vi "Patrick-UTiLIA-RollingAverage.vi"(5 "Restart Avg":bool, 6 "Current Average":dbl=0.09818164425343229 format="%.5f", 7 "Rolling Avg Parameters":T1={"Rolling Avg mode"=enum."No Averaging", "# of averages"=10} {"# of averages" min=1}, 8 "Signal to Average":dbl[](array[numeric]) format="%.2f") -> (0 "averages completed":i16, 1 "Long-term Average":dbl=0.09818164425343229 format="%.5f", 2 "Chunk Fluctuations":dbl=0.00023658579987782333 format="%.3f", 3 "Chunk Average":dbl=0.09818164425343229 format="%.5f", 4 "averaging done":bool)   [LabVIEW 2013]
uses:
  <vilib>/Analysis/NI_AALBase.lvlib
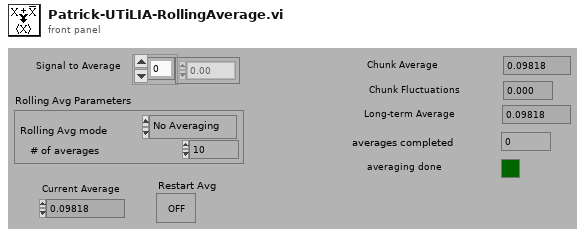
[diagram p1: front panel]
types:
  T1 = cluster{"Rolling Avg mode":enum16{"No Averaging", "Linear", "Exponential"}, "# of averages":u32}
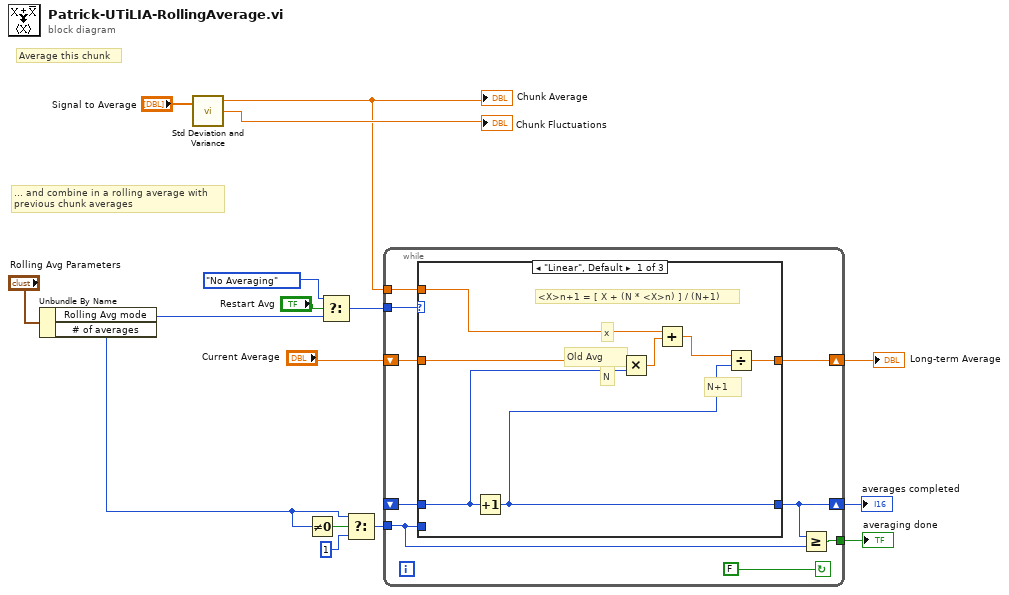
[diagram p0: block diagram]
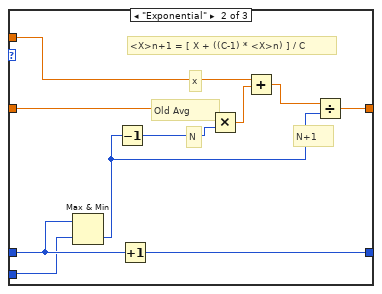
[diagram p2: hidden frame]
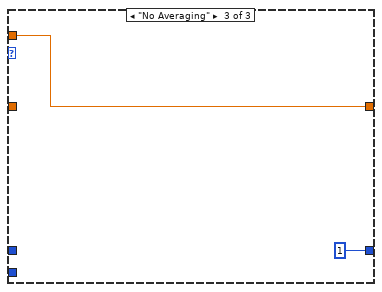
[diagram p3: hidden frame]
diagram:
  # "... and combine in a rolling average with\nprevious chunk averages"
  # "Average this chunk"
  n1 = Unbundle By Name("Rolling Avg Parameters") -> ("Rolling Avg mode"=w5:enum16{"No Averaging", "Linear", "Exponential"}, "# of averages"=w8:u32)
  n2 = call <vilib>:"Std Deviation and Variance.vi"("X"="Signal to Average") -> ("mean"=w2:dbl, "standard deviation"=→"Chunk Fluctuations":dbl)  [unwired: 1 in, 1 out]
  "Chunk Average" <- w2
  n3 = Not Equal To 0?(x=w8) -> (x != 0?=w11:bool)
  n4 = Select(t=enum16{"No Averaging", "Linear", "Exponential"}."No Averaging" ("f"), s="Restart Avg", f=w5) -> (s? t:f=w4:enum16{"No Averaging", "Linear", "Exponential"})
  n5 = Select(t=w8, s=w11, f=u32 1) -> (s? t:f=w10:u32)
  n6 = while {
    shift-right: [w25] -> w3
    shift-left: "Current Average" -> [w23]
    shift-right: [w20] -> w13
    shift-left: _ -> [w24]
    tunnel: w2 -> [w22]
    tunnel: w10 -> [w21]
    tunnel: [w19] -> w12
    tunnel: w4 -> [w17]
    stop <- FALSE continue-if-true
    n7 = case shown="\"Linear\", Default" w17 {
      tunnel: [w29 w38 w44] -> w25
      tunnel: [w27 w37 i16 1] -> w20
      tunnel: w24 -> [w26 w35 _]
      tunnel: w23 -> [w32 w40 _]
      tunnel: w22 -> [w28 w39 w44]
      tunnel: w21 -> [_ w34 _]
      frame "Linear", Default {
        # "x"
        # "Old Avg"
        # "N+1"
        # "N"
        # "<X>n+1 = [ X + (N * <X>n) ] / (N+1)"
        n8 = Increment(x=w26) -> (x+1=w27:i16)
        n9 = Multiply(x=w32, y=w26) -> (x*y=w31:dbl)
        n10 = Add(x=w28, y=w31) -> (x+y=w30:dbl)
        n11 = Divide(x=w30, y=w27) -> (x/y=w29:dbl)
      }
      frame "Exponential" {
        # "x"
        # "Old Avg"
        # "N+1"
        # "N"
        # "<X>n+1 = [ X + ((C-1) * <X>n) ] / C"
        n12 = Max & Min(x=w35, y=w34) -> (min(x,y)=w33:u32)  [unwired: 1 out]
        n13 = Decrement(x=w33) -> (x-1=w36:u32)
        n14 = Increment(x=w35) -> (x+1=w37:i16)
        n15 = Multiply(x=w40, y=w36) -> (x*y=w42:dbl)
        n16 = Add(x=w39, y=w42) -> (x+y=w41:dbl)
        n17 = Divide(x=w41, y=w33) -> (x/y=w38:dbl)
      }
      frame "No Averaging" {
      }
    }
    n18 = Greater Or Equal?(x=w20, y=w21) -> (x >= y?=w19:bool)
  }
  "Long-term Average" <- w3
  "averages completed" <- w13
  "averaging done" <- w12
